vi "main.vi"() -> ()   [LabVIEW 2011]
uses:
  ctrOWLMarker.ctl
  ctrCommonFlags.ctl
  ctrSetsFlags.ctl
  <vilib>/Platform/TimedLoop/XDataNode/timing_clust.ctl
  <vilib>/Platform/TimedLoop/XDataNode/nitl_modes.ctl
  <vilib>/Platform/TimedLoop/XDataNode/wakeup.ctl
  <vilib>/DAQmx/read.llb/DAQmx Read (Analog 2D DBL NChan NSamp).vi
  <vilib>/DAQmx/write.llb/DAQmx Write (Digital U8 1Chan 1Samp).vi
  <vilib>/DAQmx/configure/trigger.llb/DAQmx Start Trigger (Digital Edge).vi
  <vilib>/Analysis/Matrix/Numeric/Conversions/Array To Matrix - RA2.vi
  <vilib>/Analysis/baseanly.llb/Real A x B.vi
  <vilib>/Analysis/Matrix/Numeric/Conversions/Matrix To Array - RM.vi
  <vilib>/DAQmx/miscellaneous.llb/DAQmx Fill In Error Info.vi
  <vilib>/Platform/TimedLoop/XDataNode/XDataNode.xnode
  C:/Program Files/Phasespace/libowlsock.dll
  <vilib>/Platform/TimedLoop/XDataNode/XDNodeRunTimeDep.lvlib
  C:/Program Files/National Instruments/LabVIEW 2011/resource/objmgr/daqmx.rc
  <vilib>/Analysis/NI_AALBase.lvlib
  <vilib>/Analysis/Matrix/NI_Matrix.lvlib
panel:
  in  "bias transducers":bool
  in  "Calibration Files 4":path[](array[path])=[path "Z:/Yen/ATI Calib files/FT11787.cal"]
  in  "Calibration Files  3":path[](array[path])=[path "Z:/Yen/ATI Calib files/FT11332.cal"]
  in  "Calibration Files  2":path[](array[path])=[path "Z:/Yen/ATI Calib files/FT5076.cal"]
  in  "Calibration Files 1":path[](array[path])=[path "Z:/Yen/ATI Calib files/FT14967.cal"]
  out "data 4":dbl[][](array[numeric]) format="%0.2f"
  out "data 3":dbl[][](array[numeric]) format="%0.2f"
  out "data 2":dbl[][](array[numeric]) format="%0.2f"
  out "data":dbl[][](array[numeric]) format="%0.2f"
  in  "Trigger":bool
  out "markers":T1[](array[typedef])
  in  "stop":bool
  out "markers obtained (err: <0)":u16
  out "connected to server?":bool
  in  "server address":string="192.168.0.101"
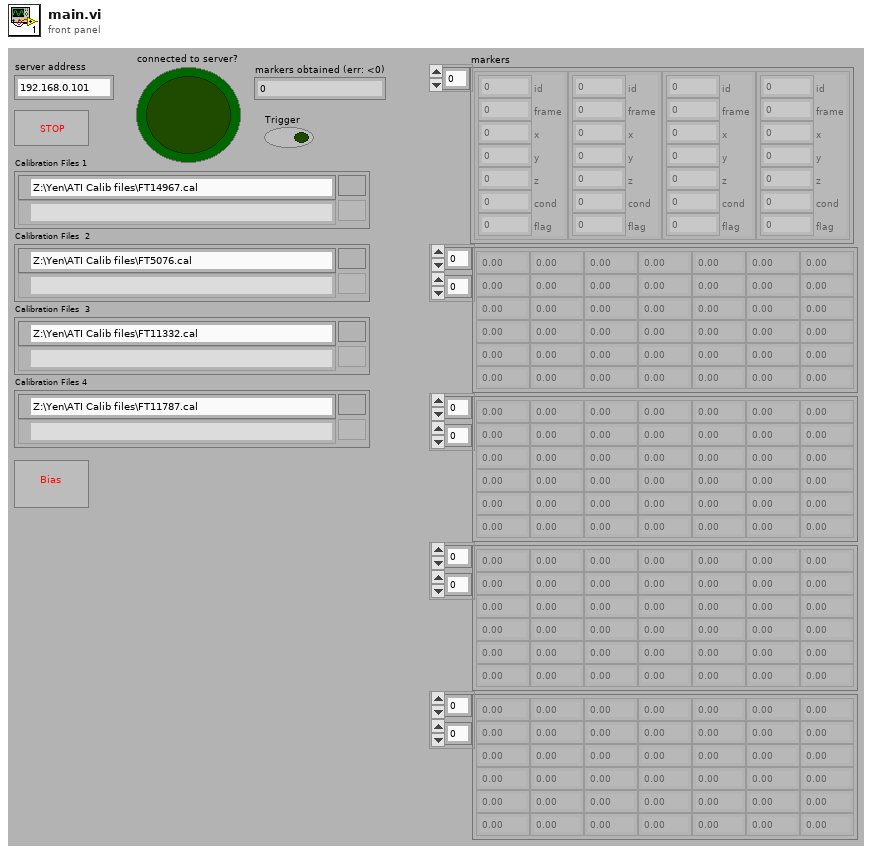
[diagram p1: front panel]
types:
  T1 = typedef "ctrOWLMarker.ctl" = cluster{"id":i32, "frame":i32, "x":sgl, "y":sgl, "z":sgl, "cond":sgl, "flag":u32}
  T2 = enum16{"open", "open or create", "create or replace", "create", "open (read-only)"}
  T3 = typedef "XDNodeRunTimeDep.lvlib/timing_clust.ctl" = cluster{"Expected End [f-1]":u64, "Actual End [f-1]":u64, "Finished Late? [f-1]":bool, "Expected End [i-1]":u64, "Actual End [i-1]":u64, "Finished Late? [i-1]":bool, "Expected Start [i]":u64, "Actual Start [i]":u64, "Expected Start [f]":u64, "Actual Start [f]":u64, "Source Name":string, "Structure Name":string, "Period":i64, "Deadline":i64, "Offset":i64, "Start":i64, "Priority":i32, "Timeout":i32, "Mode":T4, "Wakeup Reason":T5, "Error":errorcluster, "Source Type":string, "Secondary Source Type":string, "Global End Time":u64, "Global Start Time":u64, "Frame Duration":u64, "Iteration Duration":u64, "Assigned CPU":i32, "I/O Scan Engine Mode":u32}
  T4 = typedef "XDNodeRunTimeDep.lvlib/nitl_modes.ctl" = enum32{"No Change", "Process missed periods, maintain original phase", "Discard missed periods, maintain original phase", "Process missed periods, ignore original phase", "Discard missed periods, ignore original phase"}
  T5 = typedef "XDNodeRunTimeDep.lvlib/wakeup.ctl" = enum32{"Normal", "Aborted", "Asynchronous wakeup", "Timing source error", "Timed loop error", "Timeout"}
  T6 = typedef "ctrCommonFlags.ctl" = u16
  T7 = typedef "ctrSetsFlags.ctl" = u16
  T8 = typedef "NI_Matrix.lvlib/RealMatrix.ctl" = dbl[][]
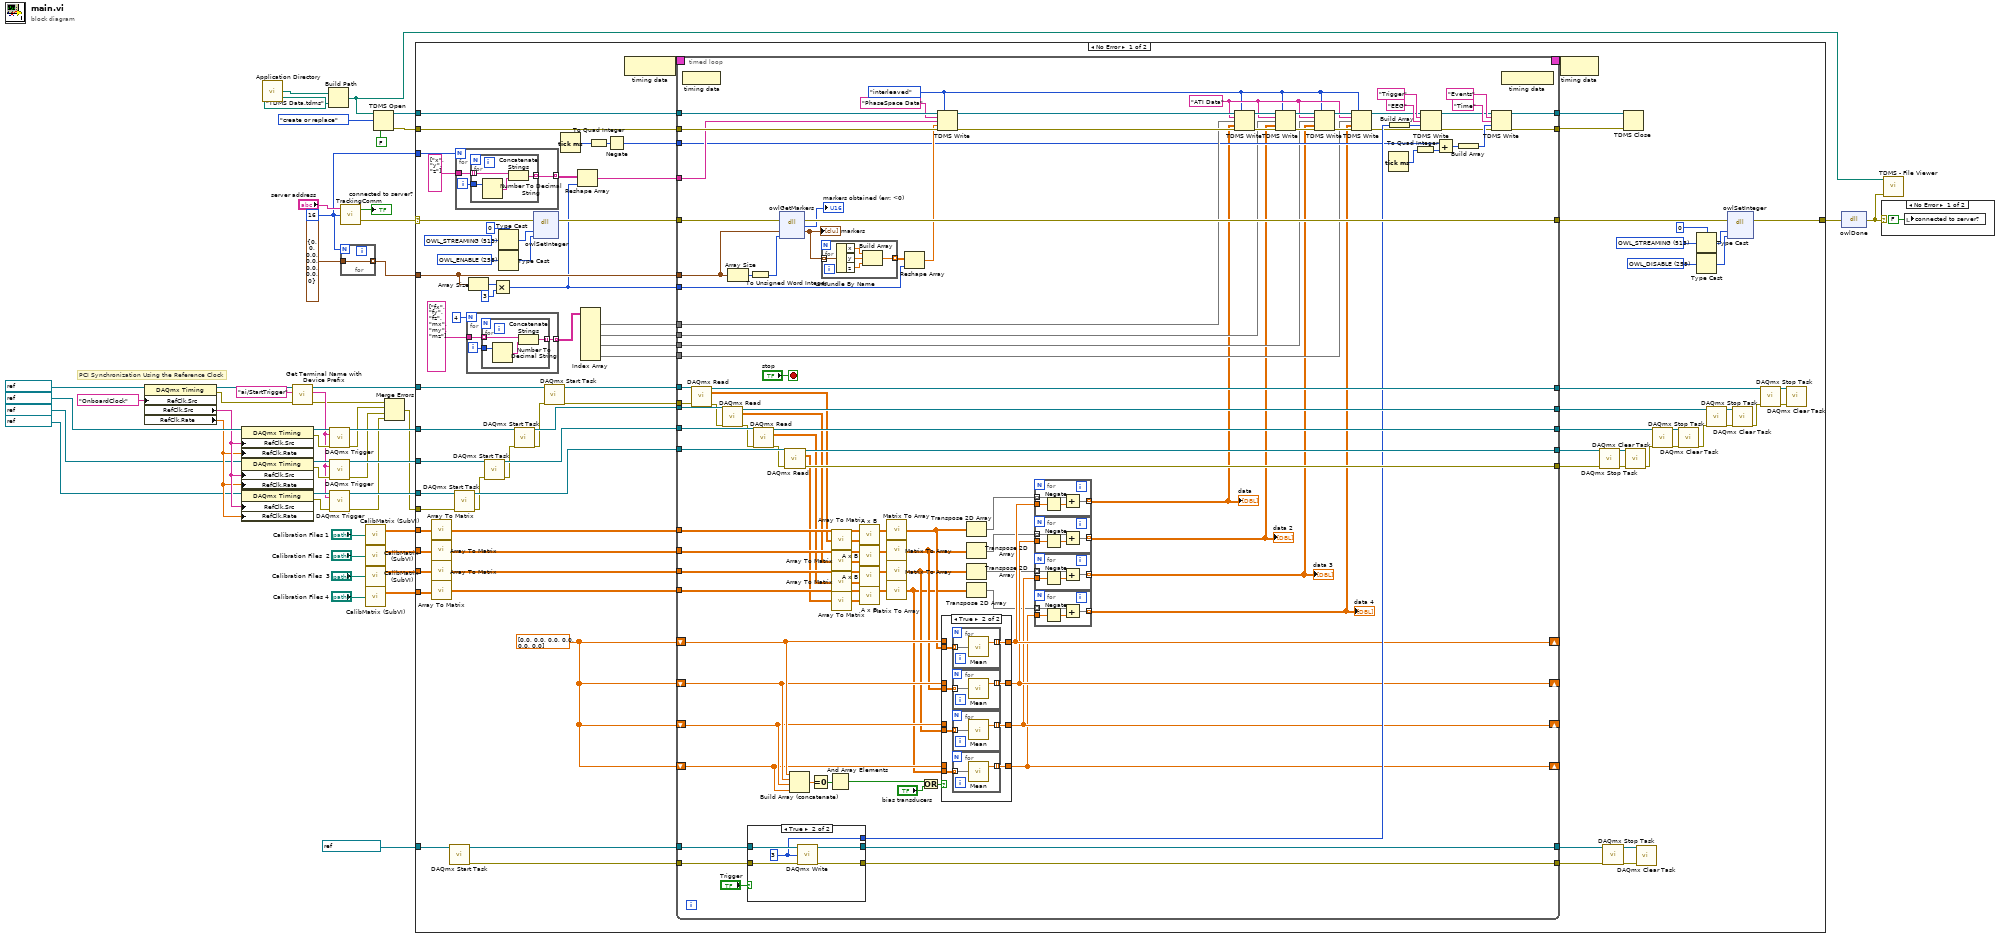
[diagram p0: block diagram]
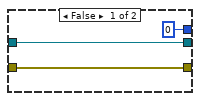
[diagram p4: hidden frame]
diagram:
  w9 = 16 ("marker tally (default: 32)")
  # "PCI Synchronization Using the Reference Clock"
  n1 = property class="DAQmx Timing"(reference=refnum<k21> "UShape1" ("DAQmx Task Name"), "RefClk.Src"=tag "OnboardClock") -> (reference out=w37:refnum<k21>, error out=w35:errorcluster, "RefClk.Src"=w41:tag, "RefClk.Rate"=w40:dbl)  [unwired: 1 in]
  n2 = property class="DAQmx Timing"(reference=refnum<k21> "UShape2" ("DAQmx Task Name"), "RefClk.Src"=w41, "RefClk.Rate"=w40) -> (reference out=w34:refnum<k21>, error out=w33:errorcluster)  [unwired: 1 in]
  n3 = property class="DAQmx Timing"(reference=refnum<k21> "UShape3" ("DAQmx Task Name"), "RefClk.Src"=w41, "RefClk.Rate"=w40) -> (reference out=w32:refnum<k21>, error out=w31:errorcluster)  [unwired: 1 in]
  n4 = property class="DAQmx Timing"(reference=refnum<k21> "UShape4" ("DAQmx Task Name"), "RefClk.Src"=w41, "RefClk.Rate"=w40) -> (reference out=w30:refnum<k21>, error out=w29:errorcluster)  [unwired: 1 in]
  n5 = call <vilib>:"Application Directory.vi"() -> ("Application Directory"=w14:path)
  n6 = call "Get Terminal Name with Device Prefix.vi"("error in (no error)"=w35, "Local Terminal Name"="ai/StartTrigger", "task/channels in"=w37) -> ("error out"=w23:errorcluster, "Terminal Name with Device Prefix"=w28:tag, "task out"=w27:refnum<k21>)  [unwired: 6 in]
  n7 = Build Path(base path=w14, name or relative path=path "TDMS Data.tdms" ("file path")) -> (appended path=w11:path)
  n8 = call-poly <vilib>:"DAQmx Trigger.vi"("task/channels in"=w34, "source"=w28, "error in"=w33) -> ("task out"=w26:refnum<k21>, "error out"=w22:errorcluster)  [unwired: 11 in]
  n9 = call-poly <vilib>:"DAQmx Trigger.vi"("task/channels in"=w32, "source"=w28, "error in"=w31) -> ("task out"=w25:refnum<k21>, "error out"=w21:errorcluster)  [unwired: 11 in]
  n10 = call-poly <vilib>:"DAQmx Trigger.vi"("task/channels in"=w30, "source"=w28, "error in"=w29) -> ("task out"=w24:refnum<k21>, "error out"=w20:errorcluster)  [unwired: 11 in]
  n11 = call "TrackingComm.vi"("marker tally (default: 32)"=w9, "server address"="server address") -> ("error out"=w48:errorcluster, "connected to server?"=→"connected to server?":bool)  [unwired: 1 in]
  n12 = for {
    N: w9 -> [_]
    tunnel: T1 {"id"=0, "frame"=0, "x"=0.0, "y"=0.0, "z"=0.0, "cond"=0.0, "flag"=0} -> [w51]
    tunnel: [w51] -> w45 mode=indexing
  }
  n13 = call "CalibMatrix (SubVI).vi"("Calibration Files"="Calibration Files 1") -> ("Calib Matrix"=w7:dbl[][])  [unwired: 1 out]
  n14 = call "CalibMatrix (SubVI).vi"("Calibration Files"="Calibration Files  2") -> ("Calib Matrix"=w6:dbl[][])  [unwired: 1 out]
  n15 = call "CalibMatrix (SubVI).vi"("Calibration Files"="Calibration Files  3") -> ("Calib Matrix"=w5:dbl[][])  [unwired: 1 out]
  n16 = call "CalibMatrix (SubVI).vi"("Calibration Files"="Calibration Files 4") -> ("Calib Matrix"=w4:dbl[][])  [unwired: 1 out]
  n17 = TDMS Open(6:FALSE ("disable buffering? (T)"), 10:T2."create or replace" ("operation"), 11:w11) -> (0:w12:errorcluster, 3:w13:refnum<k34>)  [unwired: 3 in]
  n18 = Merge Errors(w23, w22, w21, w20) -> (w19:errorcluster)
  n19 = case shown="No Error" w48 {
    selector: w48 -> [w122 w307]
    tunnel: [w134 w307] -> w47
    tunnel: w45 -> [w78 _]
    tunnel: w27 -> [w120 _]
    tunnel: w26 -> [w119 _]
    tunnel: w25 -> [w118 _]
    tunnel: w24 -> [w117 _]
    tunnel: w19 -> [w90 _]
    tunnel: refnum<k21> "TriggerDPort" ("DAQmx Task Name") -> [w89 _]
    tunnel: w13 -> [w82 _]
    tunnel: w12 -> [w81 _]
    tunnel: w9 -> [w75 _]
    tunnel: w7 -> [w60 _]
    tunnel: w6 -> [w58 _]
    tunnel: w5 -> [w57 _]
    tunnel: w4 -> [w56 _]
    frame No Error {
      w52 = dbl[] [0.0, 0.0, 0.0, 0.0, 0.0, 0.0]
      w127 = u16 0
      w124 = T6 258 items=["OWL_CREATE"=256, "OWL_DESTROY"=257, "OWL_ENABLE"=258, "OWL_DISABLE"=259] ("Common flages")
      w123 = T7 513 items=["OWL_FREQUENCY"=512, "OWL_STREAMING"=513, "OWL_INTERPOLATION"=514, "OWL_BUTTONS"=528, "OWL_MARKERS"=529, "OWL_RIGIDS"=530, "OWL_COMMDATA"=544, "OWL_TIMESTAMP"=545, "OWL_PLANES"=672, "OWL_DETECTORS"=673, "OWL_IMAGES"=674, "OWL_TRANSFORM"=49664] ("Sets flags")
      w131 = u16 0
      w132 = T6 259 items=["OWL_CREATE"=256, "OWL_DESTROY"=257, "OWL_ENABLE"=258, "OWL_DISABLE"=259] ("Common flages")
      w133 = T7 513 items=["OWL_FREQUENCY"=512, "OWL_STREAMING"=513, "OWL_INTERPOLATION"=514, "OWL_BUTTONS"=528, "OWL_MARKERS"=529, "OWL_RIGIDS"=530, "OWL_COMMDATA"=544, "OWL_TIMESTAMP"=545, "OWL_PLANES"=672, "OWL_DETECTORS"=673, "OWL_IMAGES"=674, "OWL_TRANSFORM"=49664] ("Sets flags")
      n20 = call-poly <vilib>:"Array To Matrix.vi"("Real 2D Array"=w60) -> ("Real Matrix"=w59:T8)
      n21 = call-poly <vilib>:"Array To Matrix.vi"("Real 2D Array"=w58) -> ("Real Matrix"=w55:T8)
      n22 = call-poly <vilib>:"Array To Matrix.vi"("Real 2D Array"=w57) -> ("Real Matrix"=w54:T8)
      n23 = call-poly <vilib>:"Array To Matrix.vi"("Real 2D Array"=w56) -> ("Real Matrix"=w53:T8)
      n24 = call <vilib>:"DAQmx Start Task.vi"("task/channels in"=w89) -> ("task out"=w88:refnum<k21>, "error out"=w87:errorcluster)  [unwired: 13 in]
      n25 = call <vilib>:"DAQmx Start Task.vi"("task/channels in"=w117, "error in"=w90) -> ("task out"=w113:refnum<k21>, "error out"=w101:errorcluster)  [unwired: 12 in]
      n26 = for {
        N: w75 -> [_]
        tunnel: string[] ["x", "y", "z"] -> [w144]
        tunnel: [w142] -> w73 mode=indexing
        i -> [w143]
        n27 = for {
          tunnel: w144 -> [w148] mode=indexing
          tunnel: w143 -> [w147]
          tunnel: [w145] -> w142 mode=indexing
          n28 = Number To Decimal String(number=w147) -> (decimal integer string=w146:string)  [unwired: 1 in]
          n29 = Concatenate Strings(w148, w146) -> (w145:string)
        }
      }
      n30 = for {
        N: 4 -> [_]
        tunnel: string[] ["fx", "fy", "fz", "mx", "my", "mz"] -> [w137]
        tunnel: [w135] -> w65 mode=indexing
        i -> [w136]
        n31 = for {
          tunnel: w137 -> [w141] mode=indexing
          tunnel: w136 -> [w140]
          tunnel: [w138] -> w135 mode=indexing
          n32 = Number To Decimal String(number=w140) -> (decimal integer string=w139:string)  [unwired: 1 in]
          n33 = Concatenate Strings(w141, w139) -> (w138:string)
        }
      }
      n34 = Array Size(array=w78) -> (size(s)=w77:i32)
      n35 = call <vilib>:"DAQmx Start Task.vi"("task/channels in"=w118, "error in"=w101) -> ("task out"=w114:refnum<k21>, "error out"=w100:errorcluster)  [unwired: 12 in]
      n36 = Multiply(x=w77, y=3) -> (x*y=w72:i32)
      n37 = Type Cast(type=w127, x=w123) -> (*(type *) &x=w126:u16)
      n38 = Type Cast(type=w127, x=w124) -> (*(type *) &x=w125:u16)
      n39 = call <vilib>:"DAQmx Start Task.vi"("task/channels in"=w119, "error in"=w100) -> ("task out"=w115:refnum<k21>, "error out"=w102:errorcluster)  [unwired: 12 in]
      n40 = dll-call lib="C:/Program Files/Phasespace/libowlsock.dll" fn="owlSetInteger"(error in=w122, "pname"=w126, "param"=w125) -> (error out=w121:errorcluster)  [unwired: 4 in, 2 out]
      n41 = call <vilib>:"DAQmx Start Task.vi"("task/channels in"=w120, "error in"=w102) -> ("task out"=w116:refnum<k21>, "error out"=w99:errorcluster)  [unwired: 12 in]
      n42 = Tick Count (ms)() -> (millisecond timer value=w67:u32)
      n43 = Reshape Array(w73, w72) -> (w71:string[])
      n44 = Index Array(array=w65) -> (element #1=w64:string[], element #2=w63:string[], element #3=w62:string[], element #4=w61:string[])  [unwired: 8 in]
      n45 = To Quad Integer(1:w67) -> (0:w66:i64)
      n46 = Negate(x=w66) -> (-x=w68:i64)
      n47 = node-c288() -> (w104:T3)
      n48 = timed-loop {
        tunnel: [w252] -> w128
        tunnel: w121 -> [w250]
        tunnel: w78 -> [w249]
        tunnel: w116 -> [w246]
        tunnel: w115 -> [w245]
        tunnel: w114 -> [w244]
        tunnel: w113 -> [w243]
        tunnel: [w242] -> w112
        tunnel: [w241] -> w111
        tunnel: [w240] -> w110
        tunnel: [w239] -> w109
        timing: w104 -> [_]
        timing-out: [_] -> w103
        tunnel: w99 -> [w238]
        tunnel: [w234] -> w98
        tunnel: w88 -> [w233]
        tunnel: w87 -> [w232]
        tunnel: [w231] -> w86
        tunnel: [w230] -> w84
        tunnel: w82 -> [w228]
        tunnel: w81 -> [w227]
        tunnel: [w223] -> w80
        tunnel: [w222] -> w79
        tunnel: w72 -> [w218]
        tunnel: w71 -> [w216]
        tunnel: w64 -> [w212]
        tunnel: w68 -> [w203]
        tunnel: w63 -> [w192]
        tunnel: w62 -> [w191]
        tunnel: w61 -> [w190]
        tunnel: w59 -> [w187]
        tunnel: w55 -> [w179]
        tunnel: w54 -> [w178]
        tunnel: w53 -> [w177]
        shift-right: [w164] -> _
        shift-left: w52 -> [w169]
        shift-right: [w162] -> _
        shift-left: w52 -> [w168]
        shift-right: [w161] -> _
        shift-left: w52 -> [w167]
        shift-right: [w160] -> _
        shift-left: w52 -> [w166]
        stop <- "stop" stop-if-true
        w194 = "ATI Data" ("group name")
        w193 = enum16{"decimated", "interleaved"}."interleaved" ("data layout (0:decimated)")
        n49 = node-c288() -> ()  [unwired: 1 in]
        n50 = call-poly <vilib>:"DAQmx Read.vi"("task/channels in"=w246, "error in"=w238) -> ("task out"=w242:refnum<k21>, "data"=w186:dbl[][], "error out"=w237:errorcluster)  [unwired: 11 in]
        n51 = call-poly <vilib>:"DAQmx Read.vi"("task/channels in"=w245, "error in"=w237) -> ("task out"=w241:refnum<k21>, "data"=w176:dbl[][], "error out"=w236:errorcluster)  [unwired: 11 in]
        n52 = Array Size(array=w249) -> (size(s)=w248:i32)
        n53 = case shown="True" "Trigger" {
          tunnel: w233 -> [w297 w302]
          tunnel: w232 -> [w296 w301]
          tunnel: [w297 w300] -> w231
          tunnel: [w296 w299] -> w230
          tunnel: [u8 0 ("data") w298] -> w209
          frame False {
          }
          frame True {
            w298 = u8 3 ("data")
            n54 = call-poly <vilib>:"DAQmx Write.vi"("task/channels in"=w302, "data"=w298, "error in"=w301) -> ("task out"=w300:refnum<k21>, "error out"=w299:errorcluster)  [unwired: 10 in, 1 out]
          }
        }
        n55 = To Unsigned Word Integer(number=w248) -> (unsigned 16bit integer=w251:u16)
        n56 = call-poly <vilib>:"DAQmx Read.vi"("task/channels in"=w244, "error in"=w236) -> ("task out"=w240:refnum<k21>, "data"=w175:dbl[][], "error out"=w235:errorcluster)  [unwired: 11 in]
        n57 = dll-call lib="C:/Program Files/Phasespace/libowlsock.dll" fn="owlGetMarkers"(error in=w250, "markers"=w249, "count"=w251) -> (error out=w252:errorcluster, "return type"=→"markers obtained (err: <0)":u16, "markers"=w219:T1[])  [unwired: 3 in, 1 out]
        "markers" <- w219
        n58 = call-poly <vilib>:"DAQmx Read.vi"("task/channels in"=w243, "error in"=w235) -> ("task out"=w239:refnum<k21>, "data"=w174:dbl[][], "error out"=w234:errorcluster)  [unwired: 11 in]
        n59 = Build Array (concatenate)(w169, w168, w167, w166) -> (w165:dbl[])
        n60 = Equal To 0?(x=w165) -> (x = 0?=w173:bool[])
        n61 = for {
          tunnel: w219 -> [w294] mode=indexing
          tunnel: [w290] -> w220 mode=indexing
          n62 = Unbundle By Name(w294) -> ("x"=w293:sgl, "y"=w292:sgl, "z"=w291:sgl)
          n63 = Build Array(w293, w292, w291) -> (w290:sgl[])
        }
        n64 = And Array Elements(Boolean array=w173) -> (logical AND=w170:bool)
        n65 = call-poly <vilib>:"Array To Matrix.vi"("Real 2D Array"=w186) -> ("Real Matrix"=w189:T8)
        n66 = call-poly <vilib>:"Array To Matrix.vi"("Real 2D Array"=w176) -> ("Real Matrix"=w184:T8)
        n67 = call-poly <vilib>:"Array To Matrix.vi"("Real 2D Array"=w175) -> ("Real Matrix"=w183:T8)
        n68 = call-poly <vilib>:"Array To Matrix.vi"("Real 2D Array"=w174) -> ("Real Matrix"=w180:T8)
        n69 = call-poly <vilib>:"A x B.vi"("B"=w189, "A"=w187) -> ("A x B"=w188:T8)  [unwired: 1 out]
        n70 = call-poly <vilib>:"A x B.vi"("B"=w184, "A"=w179) -> ("A x B"=w185:T8)  [unwired: 1 out]
        n71 = call-poly <vilib>:"A x B.vi"("B"=w183, "A"=w178) -> ("A x B"=w182:T8)  [unwired: 1 out]
        n72 = call-poly <vilib>:"A x B.vi"("B"=w180, "A"=w177) -> ("A x B"=w181:T8)  [unwired: 1 out]
        n73 = call-poly <vilib>:"Matrix To Array.vi"("Real Matrix"=w188) -> ("Real 2D Array"=w163:dbl[][])
        n74 = call-poly <vilib>:"Matrix To Array.vi"("Real Matrix"=w185) -> ("Real 2D Array"=w159:dbl[][])
        n75 = call-poly <vilib>:"Matrix To Array.vi"("Real Matrix"=w182) -> ("Real 2D Array"=w158:dbl[][])
        n76 = call-poly <vilib>:"Matrix To Array.vi"("Real Matrix"=w181) -> ("Real 2D Array"=w157:dbl[][])
        n77 = Reshape Array(w220, w218) -> (w215:sgl[])
        n78 = Or(x=w170, y="bias transducers") -> (x .or. y?=w171:bool)
        n79 = TDMS Write(0:w228, 1:w193, 5:"PhaseSpace Data" ("group name"), 7:w216, 9:w215, 11:w227) -> (4:w221:refnum<k34>, 15:w213:errorcluster)  [unwired: 2 out]
        n80 = case shown="True" w171 {
          tunnel: w163 -> [_ w281]
          tunnel: [w273 w280] -> w164
          tunnel: w169 -> [w273 _]
          tunnel: w159 -> [_ w279]
          tunnel: w158 -> [_ w278]
          tunnel: w157 -> [_ w277]
          tunnel: [w272 w276] -> w162
          tunnel: [w271 w275] -> w161
          tunnel: [w270 w274] -> w160
          tunnel: w168 -> [w272 _]
          tunnel: w167 -> [w271 _]
          tunnel: w166 -> [w270 _]
          frame False {
          }
          frame True {
            n81 = for {
              tunnel: w281 -> [w289] mode=indexing
              tunnel: [w288] -> w280 mode=indexing
              n82 = call <vilib>:"Mean.vi"("X"=w289) -> ("mean"=w288:dbl)  [unwired: 1 out]
            }
            n83 = for {
              tunnel: w279 -> [w287] mode=indexing
              tunnel: [w286] -> w276 mode=indexing
              n84 = call <vilib>:"Mean.vi"("X"=w287) -> ("mean"=w286:dbl)  [unwired: 1 out]
            }
            n85 = for {
              tunnel: w278 -> [w285] mode=indexing
              tunnel: [w284] -> w275 mode=indexing
              n86 = call <vilib>:"Mean.vi"("X"=w285) -> ("mean"=w284:dbl)  [unwired: 1 out]
            }
            n87 = for {
              tunnel: w277 -> [w283] mode=indexing
              tunnel: [w282] -> w274 mode=indexing
              n88 = call <vilib>:"Mean.vi"("X"=w283) -> ("mean"=w282:dbl)  [unwired: 1 out]
            }
          }
        }
        n89 = Transpose 2D Array(2D array=w163) -> (transposed array=w156:dbl[][])
        n90 = Transpose 2D Array(2D array=w159) -> (transposed array=w155:dbl[][])
        n91 = Transpose 2D Array(2D array=w158) -> (transposed array=w154:dbl[][])
        n92 = Transpose 2D Array(2D array=w157) -> (transposed array=w153:dbl[][])
        n93 = for {
          tunnel: w156 -> [w266] mode=indexing
          tunnel: w164 -> [w269]
          tunnel: [w268] -> w152 mode=indexing
          n94 = Negate(x=w269) -> (-x=w267:dbl[])
          n95 = Add(x=w266, y=w267) -> (x+y=w268:dbl[])
        }
        "data" <- w152
        n96 = for {
          tunnel: w155 -> [w262] mode=indexing
          tunnel: w162 -> [w265]
          tunnel: [w264] -> w151 mode=indexing
          n97 = Negate(x=w265) -> (-x=w263:dbl[])
          n98 = Add(x=w262, y=w263) -> (x+y=w264:dbl[])
        }
        "data 2" <- w151
        n99 = for {
          tunnel: w154 -> [w258] mode=indexing
          tunnel: w161 -> [w261]
          tunnel: [w260] -> w150 mode=indexing
          n100 = Negate(x=w261) -> (-x=w259:dbl[])
          n101 = Add(x=w258, y=w259) -> (x+y=w260:dbl[])
        }
        "data 3" <- w150
        n102 = for {
          tunnel: w153 -> [w254] mode=indexing
          tunnel: w160 -> [w257]
          tunnel: [w256] -> w149 mode=indexing
          n103 = Negate(x=w257) -> (-x=w255:dbl[])
          n104 = Add(x=w254, y=w255) -> (x+y=w256:dbl[])
        }
        "data 4" <- w149
        n105 = TDMS Write(0:w221, 1:w193, 5:w194, 7:w212, 9:w152, 11:w213) -> (4:w214:refnum<k34>, 15:w198:errorcluster)  [unwired: 2 out]
        n106 = TDMS Write(0:w214, 1:w193, 5:w194, 7:w192, 9:w151, 11:w198) -> (4:w201:refnum<k34>, 15:w197:errorcluster)  [unwired: 2 out]
        n107 = TDMS Write(0:w201, 1:w193, 5:w194, 7:w191, 9:w150, 11:w197) -> (4:w200:refnum<k34>, 15:w196:errorcluster)  [unwired: 2 out]
        n108 = TDMS Write(0:w200, 1:w193, 5:w194, 7:w190, 9:w149, 11:w196) -> (4:w199:refnum<k34>, 15:w195:errorcluster)  [unwired: 2 out]
        n109 = Tick Count (ms)() -> (millisecond timer value=w204:u32)
        n110 = Build Array(w209) -> (w208:u8[])
        n111 = To Quad Integer(1:w204) -> (0:w202:i64)
        n112 = TDMS Write(0:w199, 5:"Trigger" ("group name in (Untitled)"), 7:"EEG", 9:w208, 11:w195) -> (4:w211:refnum<k34>, 15:w210:errorcluster)  [unwired: 1 in, 2 out]
        n113 = Add(x=w203, y=w202) -> (x+y=w205:i64)
        n114 = Build Array(w205) -> (w226:i64[])
        n115 = TDMS Write(0:w211, 5:"Events" ("group name"), 7:"Time" ("channel name"), 9:w226, 11:w210) -> (4:w223:refnum<k34>, 15:w222:errorcluster)  [unwired: 1 in, 2 out]
        n116 = node-c288() -> ()  [unwired: 1 out]
      }
      n117 = node-c288(w103) -> ()
      n118 = call <vilib>:"DAQmx Stop Task.vi"("task/channels in"=w109, "error in"=w98) -> ("task out"=w105:refnum<k21>, "error out"=w97:errorcluster)  [unwired: 12 in]
      n119 = call <vilib>:"DAQmx Stop Task.vi"("task/channels in"=w86, "error in"=w84) -> ("task out"=w85:refnum<k21>, "error out"=w83:errorcluster)  [unwired: 12 in]
      n120 = TDMS Close(8:w79, 11:w80) -> ()  [unwired: 2 out]
      n121 = call <vilib>:"DAQmx Clear Task.vi"("task in"=w105, "error in"=w97) -> ("error out"=w96:errorcluster)  [unwired: 13 in]
      n122 = call <vilib>:"DAQmx Clear Task.vi"("task in"=w85, "error in"=w83) -> ()  [unwired: 13 in, 1 out]
      n123 = call <vilib>:"DAQmx Stop Task.vi"("task/channels in"=w110, "error in"=w96) -> ("task out"=w106:refnum<k21>, "error out"=w95:errorcluster)  [unwired: 12 in]
      n124 = call <vilib>:"DAQmx Clear Task.vi"("task in"=w106, "error in"=w95) -> ("error out"=w94:errorcluster)  [unwired: 13 in]
      n125 = Type Cast(type=w131, x=w133) -> (*(type *) &x=w130:u16)
      n126 = Type Cast(type=w131, x=w132) -> (*(type *) &x=w129:u16)
      n127 = call <vilib>:"DAQmx Stop Task.vi"("task/channels in"=w111, "error in"=w94) -> ("task out"=w107:refnum<k21>, "error out"=w93:errorcluster)  [unwired: 12 in]
      n128 = dll-call lib="C:/Program Files/Phasespace/libowlsock.dll" fn="owlSetInteger"(error in=w128, "pname"=w130, "param"=w129) -> (error out=w134:errorcluster)  [unwired: 4 in, 2 out]
      n129 = call <vilib>:"DAQmx Clear Task.vi"("task in"=w107, "error in"=w93) -> ("error out"=w92:errorcluster)  [unwired: 13 in]
      n130 = call <vilib>:"DAQmx Stop Task.vi"("task/channels in"=w112, "error in"=w92) -> ("task out"=w108:refnum<k21>, "error out"=w91:errorcluster)  [unwired: 12 in]
      n131 = call <vilib>:"DAQmx Clear Task.vi"("task in"=w108, "error in"=w91) -> ()  [unwired: 13 in, 1 out]
    }
    frame Error {
    }
  }
  n132 = dll-call lib="C:/Program Files/Phasespace/libowlsock.dll" fn="owlDone"(error in=w47) -> (error out=w10:errorcluster)  [unwired: 2 in, 2 out]
  n133 = case shown="No Error" w10 {
    frame No Error {
      n134 = local write "connected to server?"(FALSE) -> ()
    }
    frame Error {
    }
  }
  n135 = call <vilib>:"TDMS - File Viewer.vi"("error in (no error)"=w10, "file path"=w11) -> ()  [unwired: 6 out]
